vi "Uncircumcise Lock-in .vi"() -> ()   [LabVIEW 2015]
uses:
  <vilib>/measure/matone.llb/Extract Single Tone Information 1 Chan.vi
  <vilib>/measure/NI_MAPro.lvlib
panel:
  out "Waveform Graph 2":waveform(dbl)(graph)
  in  "Save result":bool
  out "detected phase (deg)":dbl format="%#_20p"
  out "XY Graph":cluster{dbl[], "Y":dbl[]}[](graph)
  in  "Phase shift":dbl=134.0
  in  "Clip units of Ts off":dbl
  in  "Filter type":enum16{"None", "IIR", "FIR"}(ring)=enum."IIR"
  in  "Fix time delay":bool=TRUE
  in  "Time constant":dbl=0.0001 format="%#_6p"
  out "detected frequency":dbl format="%#_20p"
  out "Waveform Graph":waveform(dbl)[](graph)
  in  "Input file":path
  in  "Reference channel":string="IL2"
  in  "Signal channel":string="VL2"
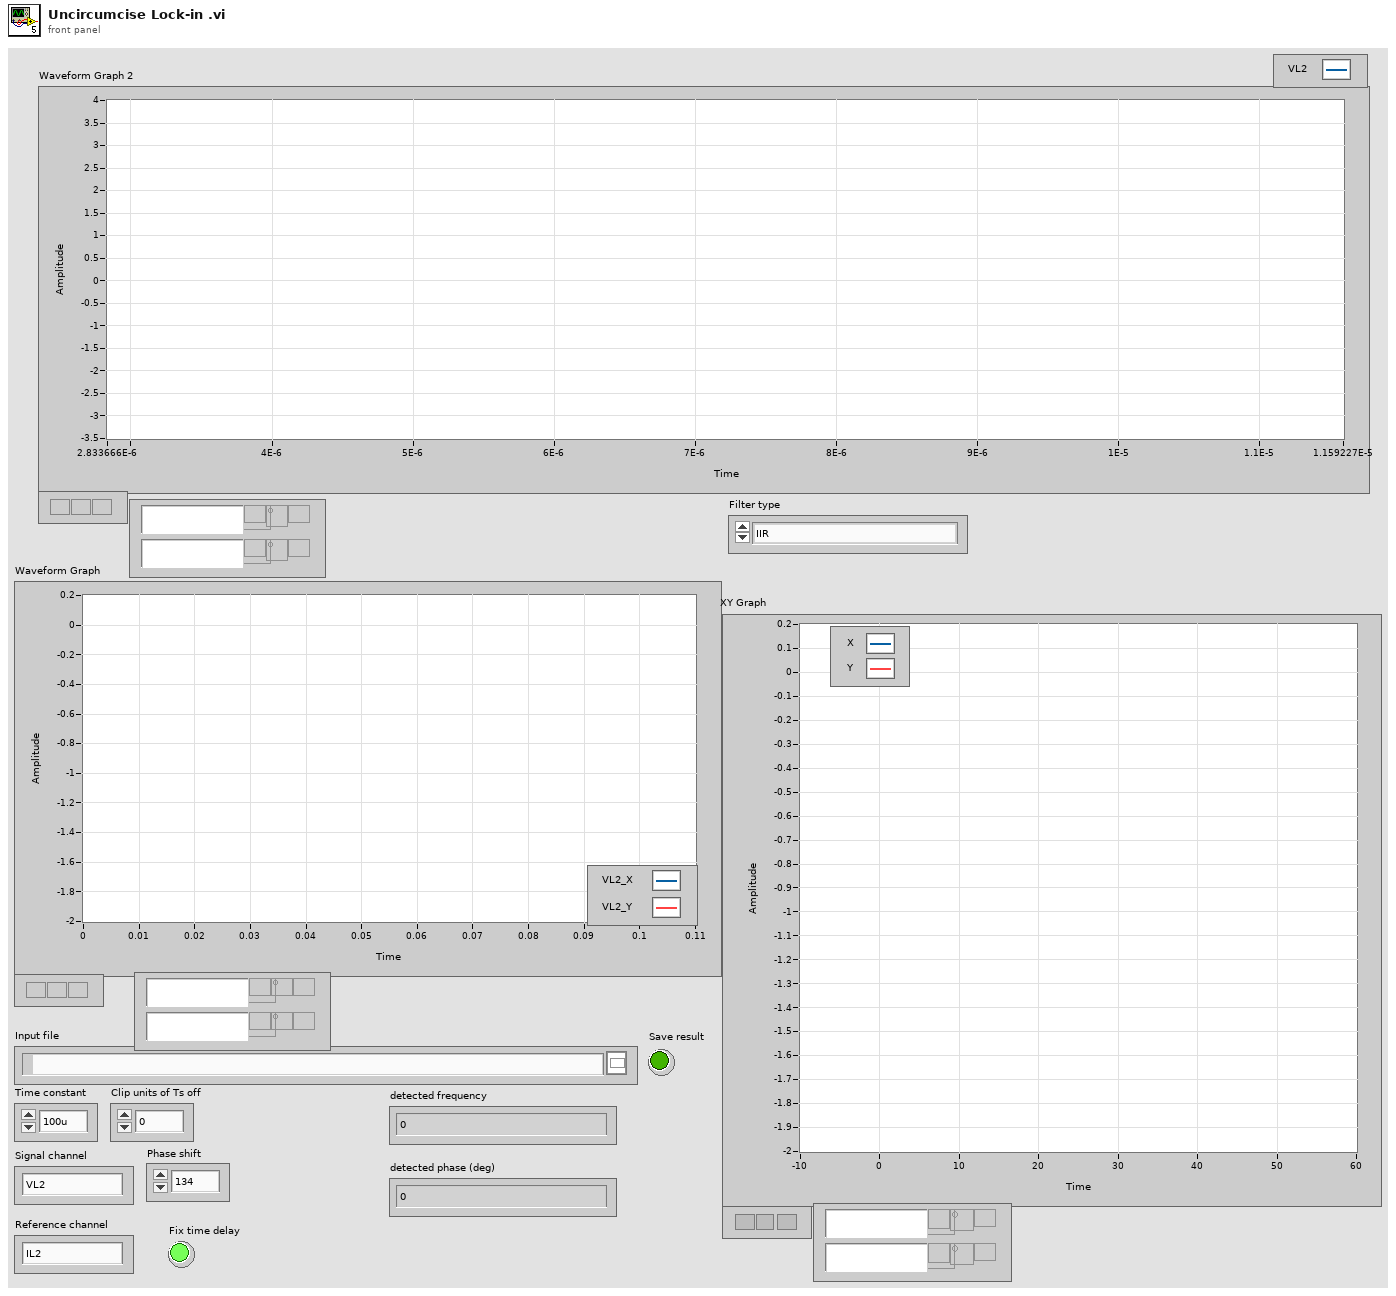
[diagram p1: front panel]
types:
  T1 = enum16{"open", "open or create", "create or replace", "create", "open (read-only)"}
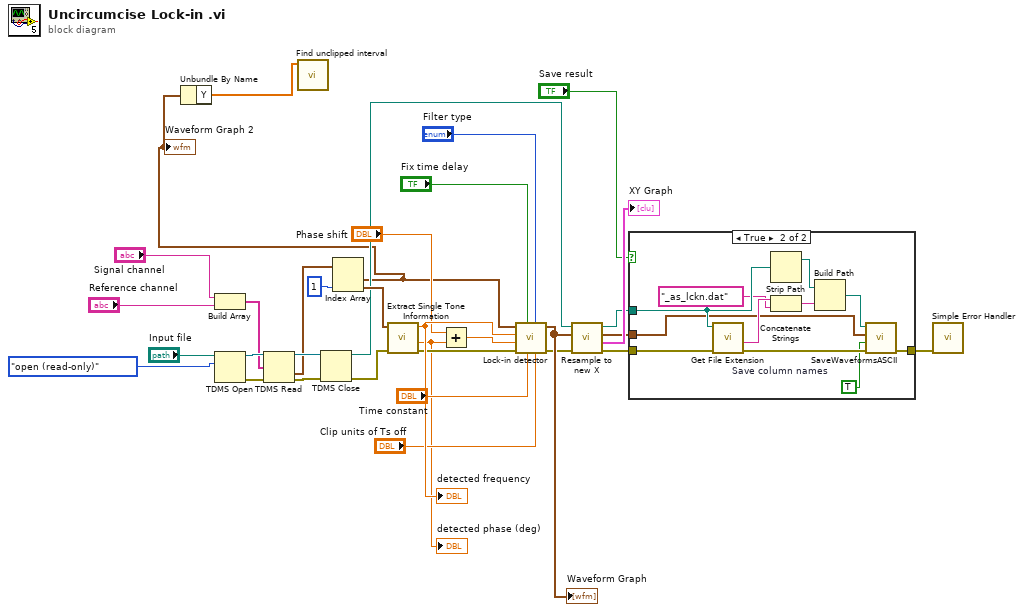
[diagram p0: block diagram]
diagram:
  n1 = Build Array("Signal channel", "Reference channel") -> (w27:string[])
  n2 = TDMS Open(10:T1."open (read-only)" ("operation (0:open)"), 11:"Input file") -> (0:w30:errorcluster, 3:w31:refnum<k34>)  [unwired: 5 in]
  n3 = TDMS Read(0:w31, 7:w27, 11:w30) -> (4:w26:refnum<k34>, 10:w24:waveform(dbl)[], 15:w25:errorcluster)  [unwired: 5 in, 3 out]
  n4 = TDMS Close(8:w25, 11:w26) -> (0:w19:errorcluster, 3:w11:path)
  n5 = Index Array(array=w24, index #2=1 ("index")) -> (element #1=w2:waveform(dbl), element #2=w22:waveform(dbl))  [unwired: 1 in]
  "Waveform Graph 2" <- w2
  n6 = Unbundle By Name(w2) -> ("Y"=w1:dbl[])
  n7 = call "Find unclipped interval.vi"("Data"=w1) -> ()  [unwired: 11 in]
  n8 = call-poly <vilib>:"Extract Single Tone Information.vi"("error in (no error)"=w19, "time signal in"=w22) -> ("error out"=w20:errorcluster, "detected phase (deg)"=w8:dbl, "detected frequency"=w21:dbl)  [unwired: 4 in, 3 out]
  "detected frequency" <- w21
  "detected phase (deg)" <- w8
  n9 = Add(x="Phase shift", y=w8) -> (x+y=w14:dbl)
  n10 = call "Lock-in detector.vi"("Clip units of Ts off"="Clip units of Ts off", "Filter type"="Filter type", "Time constant"="Time constant", "Fix time delay"="Fix time delay", "Error In"=w20, "Phase"=w14, "Frequency"=w21, "Data in"=w2) -> ("Error Out"=w10:errorcluster, "Data out"=w12:waveform(dbl)[])  [unwired: 2 in]
  "Waveform Graph" <- w12
  n11 = call "Resample to new X.vi"("Error In"=w10, "Signal"=w12, "X-axis file"=w11) -> ("Error Out"=w5:errorcluster, "XY Graph"=→"XY Graph":cluster{dbl[], "Y":dbl[]}[], "Resampled Signal"=w6:waveform(dbl)[], "X-axis file out"=w7:path)  [unwired: 5 in]
  n12 = case shown="True" "Save result" {
    tunnel: w7 -> [_ w45]
    tunnel: w6 -> [_ w40]
    tunnel: w5 -> [w34 w37]
    tunnel: [w34 w36] -> w3
    frame False {
    }
    frame True {
      w35 = TRUE  # Save column names
      n13 = call <vilib>:"Get File Extension.vi"("error in (no error)"=w37, "file"=w45) -> ("error out"=w38:errorcluster, "filename without extension"=w44:string)  [unwired: 5 in, 3 out]
      n14 = Strip Path(path=w45) -> (stripped path=w42:path)  [unwired: 1 out]
      n15 = Concatenate Strings(w44, "_as_lckn.dat" ("string")) -> (w41:string)
      n16 = Build Path(base path=w42, name or relative path=w41) -> (appended path=w39:path)
      n17 = call "SaveWaveformsASCII.vi"("error in"=w38, "Save column names"=w35, "waveforms in"=w40, "file (use dialog)"=w39) -> ("error out"=w36:errorcluster)  [unwired: 7 in]
    }
  }
  n18 = call <vilib>:"Simple Error Handler.vi"("error in (no error)"=w3) -> ()  [unwired: 4 in, 5 out]
